vi "sub_PSKMod_Temp.vi"(0 "Packet to Transmit":i8[](array[numeric]), 2 "PSK system parameters":T2 {"PSK type" items=["normal", "shifted", "offset"]; "symbol map" format="%.3f"}, 7 "Symbol Rate, Hz":dbl=1.0 format="%.2f", 11 "error in (no error)":errorcluster, 12 "filter parameters":T1={"Alpha"=0.5, "Filter Length"=6, "TX Filter"=enum."Root Raised Cos"} {"Alpha" format="%.2f"}) -> (4 "output complex waveform":cluster{"t0":dbl, "dt":dbl, "Y":cdb[]} {"Y" format="%.3f"; "dt" format="%^.2e"; "t0" format="%.4f"}, 8 "samples per symbol":i32, 15 "error out":errorcluster)   [LabVIEW 2023]
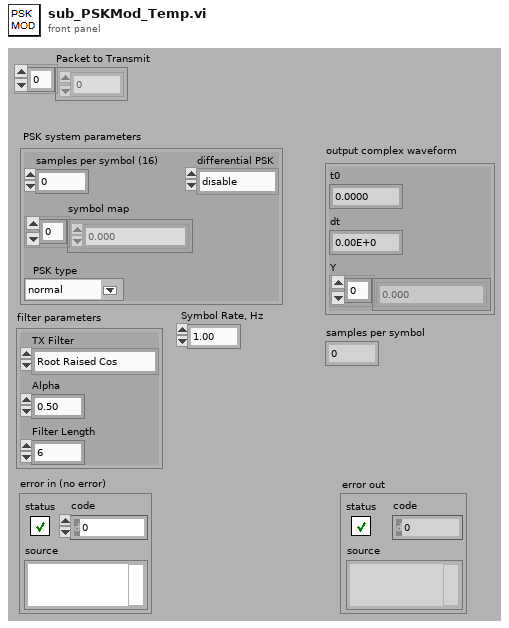
[diagram p1: front panel]
types:
  T1 = cluster{"Alpha":dbl, "Filter Length":i32, "TX Filter":enum16{"none", "Raised Cosine", "Root Raised Cos", "Gaussian"}}
  T2 = cluster{"samples per symbol (16)":i32, "symbol map":cdb[], "differential PSK":enum16{"disable", "enable"}, "PSK type":u16}
  T3 = enum16{"FSK", "PSK", "QAM", "MSK", "PAM", "ASK", "CPM"}
  T4 = typedef "niAMT.lvlib/Complex Data Waveform.ctl" = cluster{"t0":dbl, "dt":dbl, "Y":cdb[]}
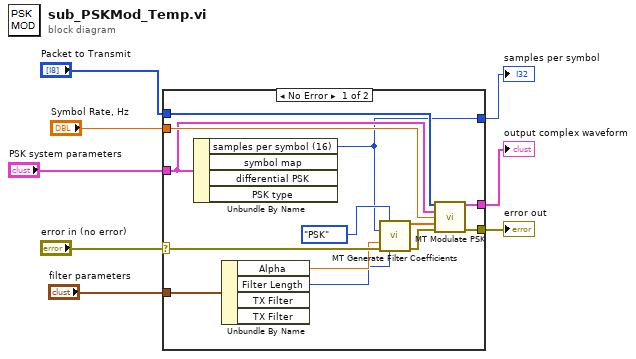
[diagram p0: block diagram]
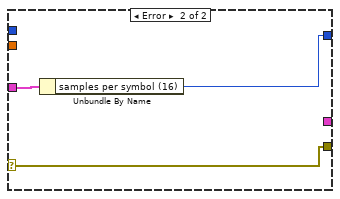
[diagram p2: hidden frame]
diagram:
  n1 = case shown="No Error" "error in (no error)" {
    selector: "error in (no error)" -> [w21 w24]
    tunnel: [w19 w24] -> w8
    tunnel: "Symbol Rate, Hz" -> [w16 _]
    tunnel: "PSK system parameters" -> [w12 w23]
    tunnel: "filter parameters" -> [w17 _]
    tunnel: "Packet to Transmit" -> [w18 _]
    tunnel: [w15 _] -> w2
    tunnel: [w9 w22] -> w1
    frame No Error {
      n2 = Unbundle By Name(w12) -> ("samples per symbol (16)"=w9:i32)  [unwired: 3 out]
      n3 = Unbundle By Name(w17) -> ("Alpha"=w14:dbl, "Filter Length"=w13:i32)  [unwired: 2 out]
      n4 = call <vilib>:"MT Generate Filter Coefficients.vi"("modulation type"=T3."PSK", "pulse shaping samples per symbol (16)"=w9, "filter parameter"=w14, "error in (no error)"=w21, "filter length (symbols)"=w13) -> ("pulse shaping filter coefficients"=w10:dbl[], "error out"=w20:errorcluster)  [unwired: 8 in, 1 out]
      n5 = call <vilib>:"MT Modulate PSK.vi"("input bit stream"=w18, "PSK system parameters"=w12, "symbol rate (Hz)"=w16, "pulse shaping filter coefficients"=w10, "error in (no error)"=w20) -> ("output complex waveform"=w15:T4, "error out"=w19:errorcluster)  [unwired: 8 in, 1 out]
    }
    frame Error {
      n6 = Unbundle By Name(w23) -> ("samples per symbol (16)"=w22:i32)
    }
  }
  "error out" <- w8
  "output complex waveform" <- w2
  "samples per symbol" <- w1
